vi "Periodic Tasks.vi"(8 "error in":errorcluster) -> ()   [LabVIEW 2023]
doc: "This VI runs in parallel to other tasks. It can contain as many user-defined periodic loops as you need. These can carry out PID or other sorts of timed response."
uses:
  <vilib>/Rock Robotics/WPI/DriverStation/WPI_DriverStationAllianceInfo.ctl
  <vilib>/Rock Robotics/Network Tables/NT Read String.vi
  <vilib>/Rock Robotics/Network Tables/NT Write String.vi
  GeneralPurpose/AllianceColorGlobal.vi
  <vilib>/Rock Robotics/WPI/ThirdParty/PhotonVisionLib/PhotonVisionLib.lvlib
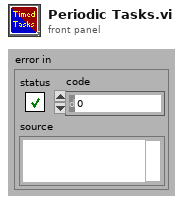
[diagram p1: front panel]
types:
  T1 = typedef "WPI_DriverStationAllianceInfo.ctl" = enum16{"Red", "Blue", "Invalid"}
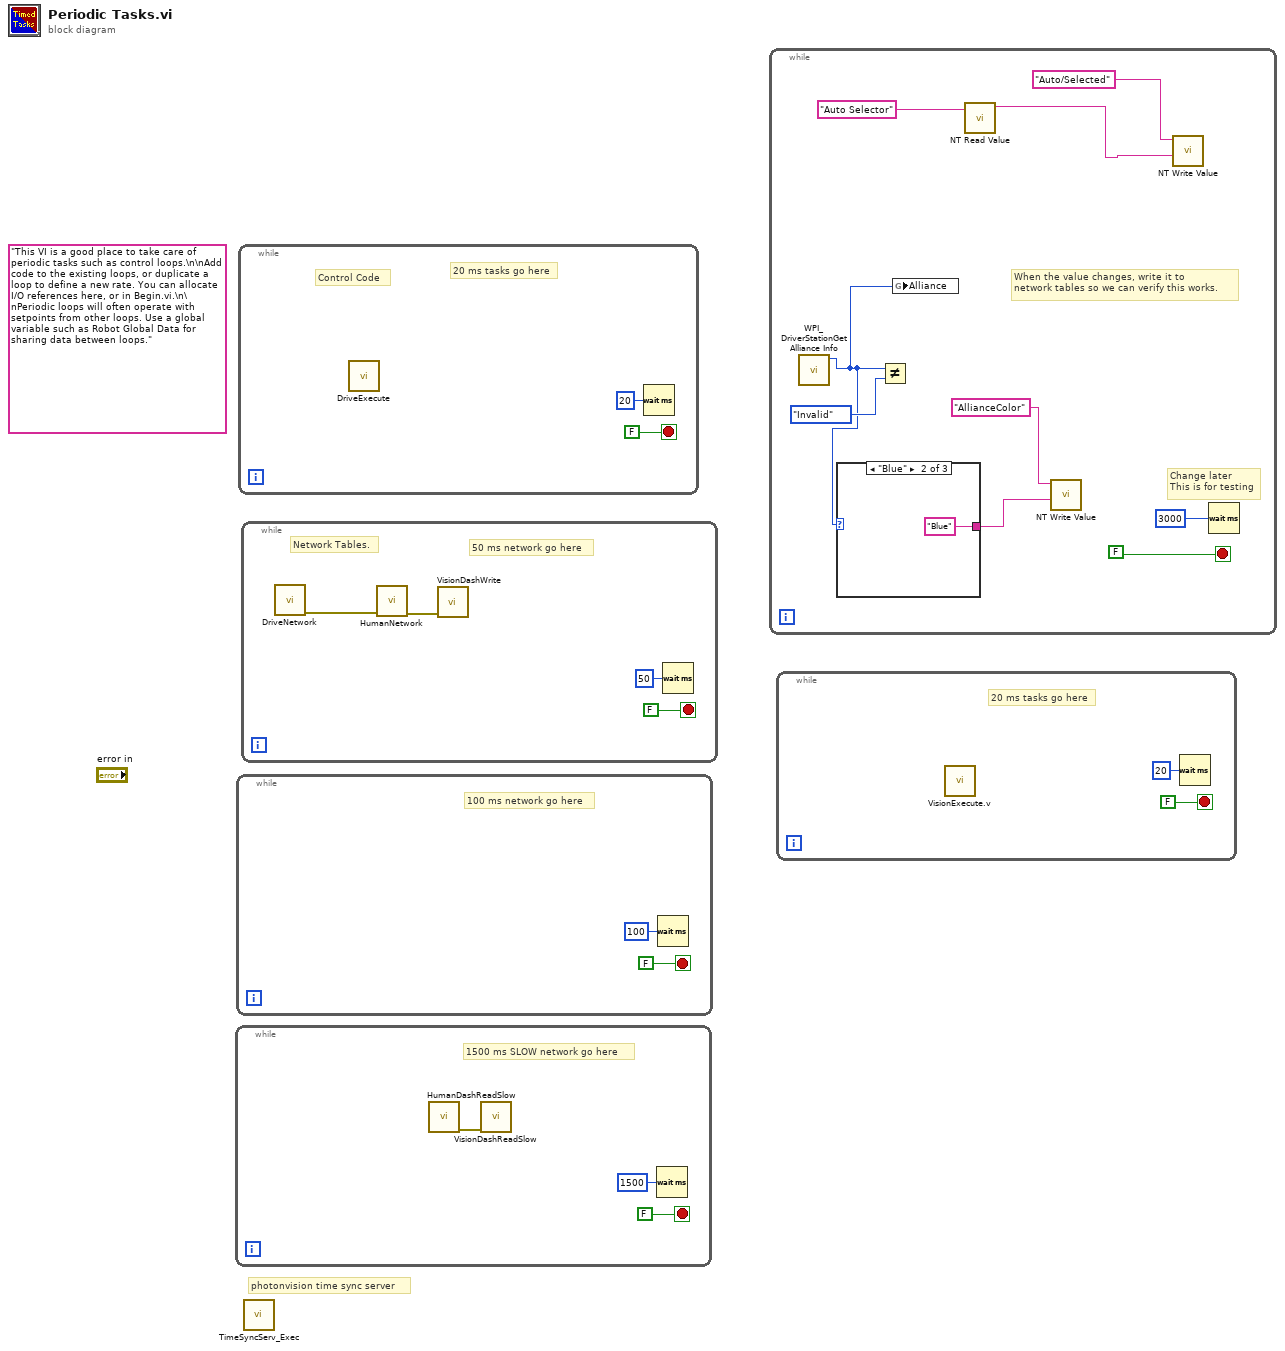
[diagram p0: block diagram]
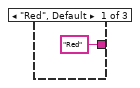
[diagram p2: hidden frame]
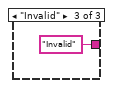
[diagram p3: hidden frame]
diagram:
  (unwired) "This VI is a good place to take care of periodic tasks such as control loops.\n\nAdd code to the existing loops, or duplicate a loop to define a new rate. You can allocate I/O references here, or in Begin.vi.\n\nPeriodic loops will often operate with setpoints from other loops. Use a global variable such as Robot Global Data for sharing data between loops."
  # "photonvision time sync server"
  n1 = while {
    stop <- FALSE stop-if-true
    # "1500 ms SLOW network go here"
    n2 = call "HumanDashReadSlow.vi"() -> ("error out"=w1:errorcluster)  [unwired: 11 in]
    n3 = call "VisionDashReadSlow.vi"("error in (no error)"=w1) -> ()  [unwired: 10 in, 1 out]
    n4 = Wait (ms)(milliseconds to wait=u32 1500) -> ()  [unwired: 1 out]
  }
  n5 = while {
    stop <- FALSE stop-if-true
    # "100 ms network go here"
    n6 = Wait (ms)(milliseconds to wait=u32 100) -> ()  [unwired: 1 out]
  }
  n7 = while {
    stop <- FALSE stop-if-true
    # "Control Code"
    # "20 ms tasks go here"
    n8 = call "DriveExecute.vi"() -> ()  [unwired: 11 in, 1 out]
    n9 = Wait (ms)(milliseconds to wait=u32 20) -> ()  [unwired: 1 out]
  }
  n10 = while {
    stop <- FALSE stop-if-true
    # "Network Tables."
    # "50 ms network go here"
    n11 = call "DriveNetwork.vi"() -> ("error out"=w8:errorcluster)  [unwired: 11 in]
    n12 = call "HumanNetwork.vi"("error in (no error)"=w8) -> ("error out"=w9:errorcluster)  [unwired: 10 in]
    n13 = call "VisionDashWrite.vi"("error in (no error)"=w9) -> ()  [unwired: 10 in, 1 out]
    n14 = Wait (ms)(milliseconds to wait=u32 50) -> ()  [unwired: 1 out]
  }
  n15 = call <vilib>:"TimeSyncServ_Exec.vi"() -> ()  [unwired: 12 in]
  n16 = while {
    stop <- FALSE stop-if-true
    # "When the value changes, write it to \nnetwork tables so we can verify this works."
    # "Change later\nThis is for testing"
    n17 = call <vilib>:"WPI_DriverStationGet Alliance Info.vi"() -> ("Alliance"=w17:T1)  [unwired: 6 in, 5 out]
    n18 = case shown="\"Blue\"" w17 {
      tunnel: ["Red" "Blue" "Invalid"] -> w16
      frame "Red", Default {
      }
      frame "Blue" {
      }
      frame "Invalid" {
      }
    }
    n19 = Not Equal?(x=w17, y=WPI_DriverStationAllianceInfo."Invalid") -> ()  [unwired: 1 out]
    n20 = global write "AllianceColorGlobal.vi" "Alliance"(w17) -> ()
    n21 = call-poly <vilib>:"NT Read Value.vi"("name"="Auto Selector" ("Name")) -> ("value"=w12:string)  [unwired: 8 in, 2 out]
    n22 = call-poly <vilib>:"NT Write Value.vi"("value"=w16, "name"="AllianceColor") -> ()  [unwired: 9 in, 1 out]
    n23 = call-poly <vilib>:"NT Write Value.vi"("value"=w12, "name"="Auto/Selected") -> ()  [unwired: 9 in, 1 out]
    n24 = Wait (ms)(milliseconds to wait=u32 3000) -> ()  [unwired: 1 out]
  }
  n25 = while {
    stop <- FALSE stop-if-true
    # "20 ms tasks go here"
    n26 = call "VisionExecute.v.vi"() -> ()  [unwired: 12 in]
    n27 = Wait (ms)(milliseconds to wait=u32 20) -> ()  [unwired: 1 out]
  }
